vi "processCanFrame.vi"(1 "frame IN":u8[](array[numeric])) -> (0 "stateOut":enum16{"unconn", "reciving", "disconn"}(ring)=enum."reciving")   [LabVIEW 2021]
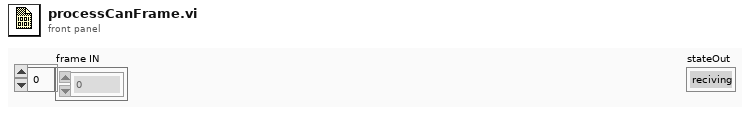
[diagram p1: front panel]
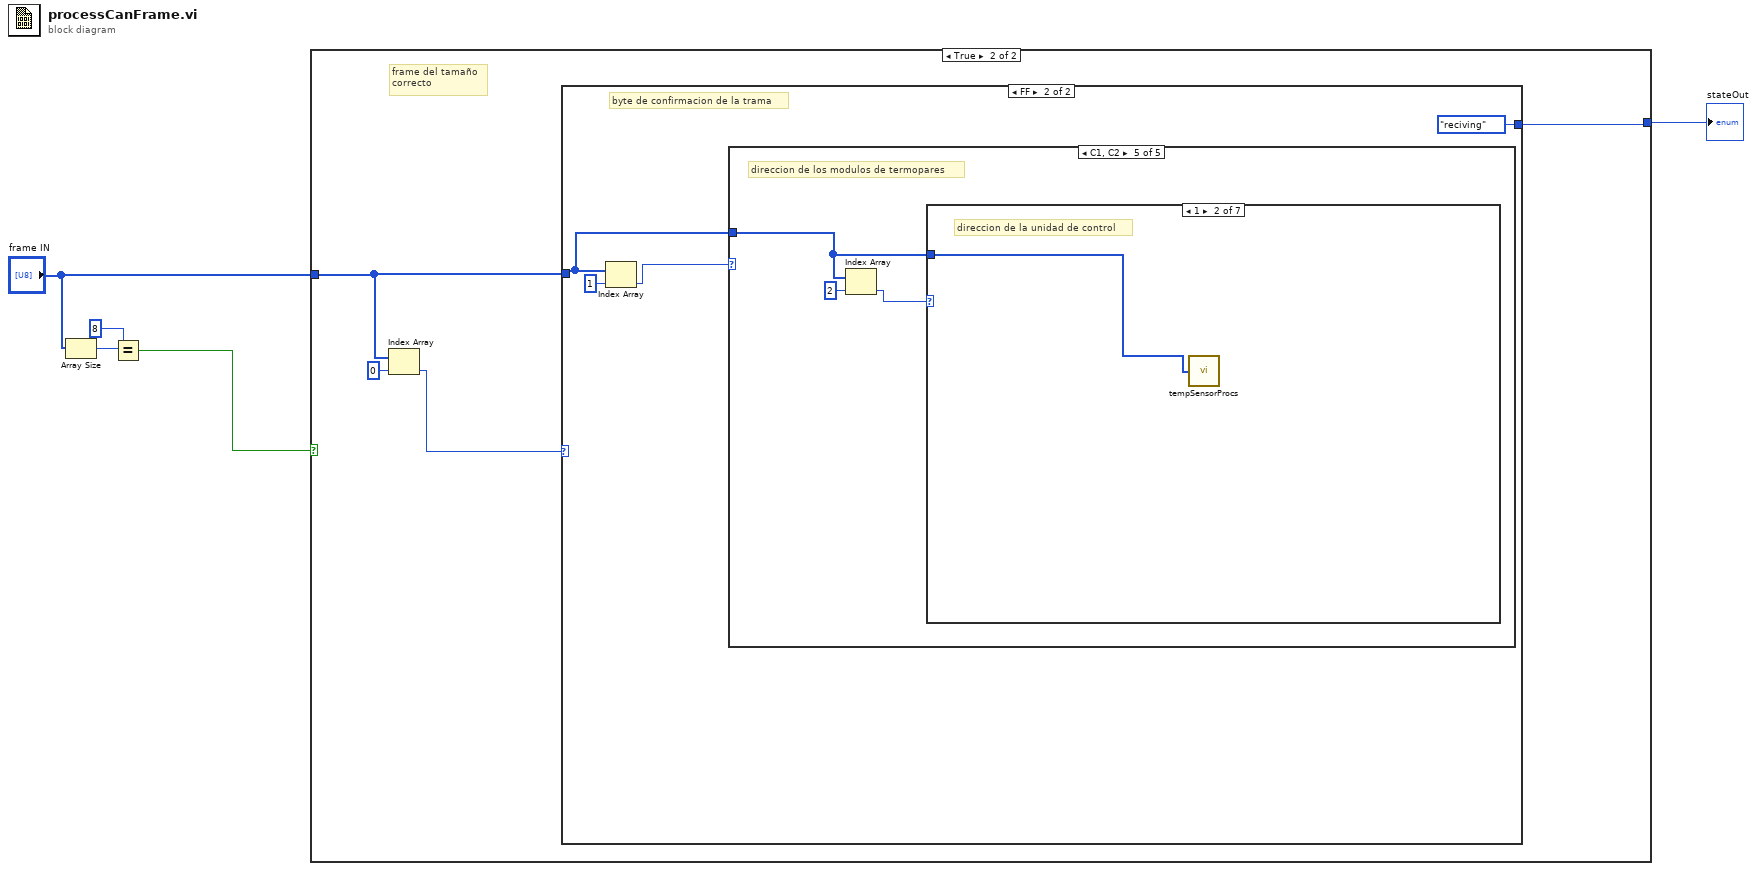
[diagram p0: block diagram]
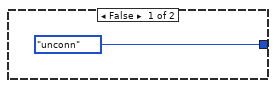
[diagram p2: hidden frame]
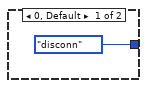
[diagram p3: hidden frame]
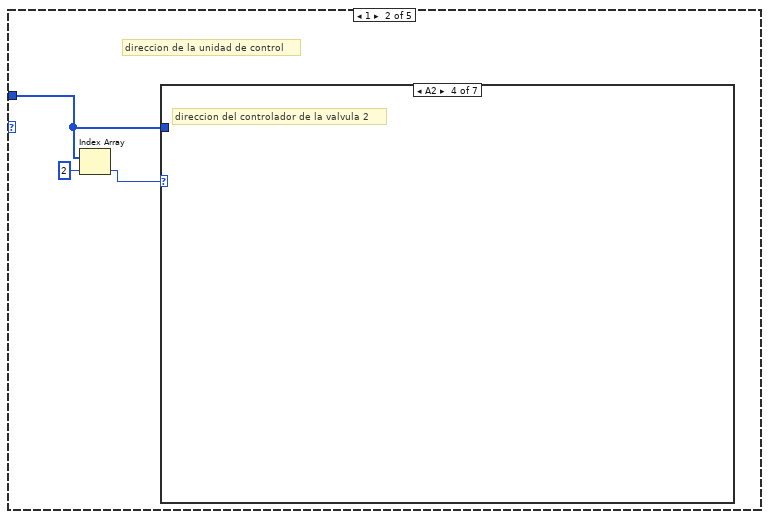
[diagram p5: hidden frame]
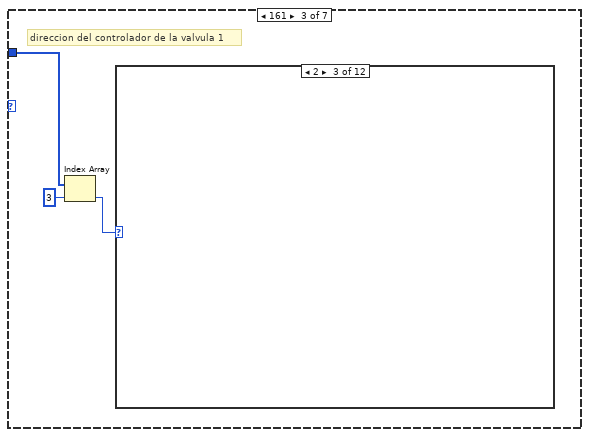
[diagram p8: hidden frame]
diagram:
  n1 = Array Size(array="frame IN") -> (size(s)=w4:i32)
  n2 = Equal?(x=w4, y=8) -> (x = y?=w2:bool)
  n3 = case shown="True" w2 {
    tunnel: "frame IN" -> [_ w9]
    tunnel: [enum16{"unconn", "reciving", "disconn"}."unconn" w7] -> w1
    frame False {
    }
    frame True {
      # "frame del tamaño\ncorrecto"
      n4 = Index Array(array=w9, index=0) -> (element=w8:u8)
      n5 = case shown="FF" w8 {
        tunnel: w9 -> [_ w13]
        tunnel: [enum16{"unconn", "reciving", "disconn"}."disconn" enum16{"unconn", "reciving", "disconn"}."reciving"] -> w7
        frame 0, Default {
        }
        frame 255 {
          # "byte de confirmacion de la trama"
          n6 = Index Array(array=w13, index=1) -> (element=w14:u8)
          n7 = case shown="C1, C2" w14 {
            tunnel: w13 -> [_ w16 w22 w29 w33]
            frame 0, Default {
            }
            frame 1 {
              # "direccion de la unidad de control"
              n8 = Index Array(array=w16, index=2) -> (element=w17:u8)
              n9 = case shown="A2" w17 {
                tunnel: w16 -> [_ _ w20 _ _ _ _]
                frame 0, Default {
                }
                frame 1 {
                  # "direccion de la unidad de control"
                }
                frame 161 {
                  # "direccion del controlador de la valvula 1"
                  n10 = Index Array(array=w20, index=3) -> (element=w19:u8)
                  n11 = case shown="2" w19 {
                    frame 0 {
                    }
                    frame 1 {
                    }
                    frame 2 {
                    }
                    frame 3 {
                    }
                    frame 4 {
                    }
                    frame 5 {
                    }
                    frame 6 {
                    }
                    frame 7 {
                    }
                    frame 8 {
                    }
                    frame 9 {
                    }
                    frame 10 {
                    }
                    frame 11, Default {
                    }
                  }
                }
                frame 162 {
                  # "direccion del controlador de la valvula 2"
                }
                frame 177 {
                  # "direccion del modulo de sensores de presion"
                }
                frame 193 {
                  # "direccion del modulo de termopares 1"
                }
                frame 194 {
                  # "direccion del modulo de termopares 2"
                }
              }
            }
            frame 161, 162 {
              # "direccion de los controladores de las valvulas"
              n12 = Index Array(array=w22, index=2) -> (element=w23:u8)
              n13 = case shown="1" w23 {
                tunnel: w22 -> [_ w25 _ _ _ _ _]
                frame 0, Default {
                }
                frame 1 {
                  # "direccion de la unidad de control"
                  n14 = Index Array(array=w25, index=3) -> (element=w26:u8)
                  n15 = case shown="4" w26 {
                    tunnel: w25 -> [_ w28]
                    frame 0, Default {
                    }
                    frame 4 {
                      n16 = call "valveDataProc.vi"("frame"=w28) -> ()
                    }
                  }
                }
                frame 161 {
                  # "direccion del controlador de la valvula 1"
                }
                frame 162 {
                  # "direccion del controlador de la valvula 2"
                }
                frame 177 {
                  # "direccion del modulo de sensores de presion"
                }
                frame 193 {
                  # "direccion del modulo de termopares 1"
                }
                frame 194 {
                  # "direccion del modulo de termopares 2"
                }
              }
            }
            frame 177 {
              # "direccion del modulo de sensores de presion"
              n17 = Index Array(array=w29, index=2) -> (element=w30:u8)
              n18 = case shown="1" w30 {
                tunnel: w29 -> [_ w32 _ _ _ _ _]
                frame 0, Default {
                }
                frame 1 {
                  # "direccion de la unidad de control"
                  n19 = call "pressSensorLin.vi"("frame"=w32) -> ()
                }
                frame 161 {
                  # "direccion del controlador de la valvula 1"
                }
                frame 162 {
                  # "direccion del controlador de la valvula 2"
                }
                frame 177 {
                  # "direccion del modulo de sensores de presion"
                }
                frame 193 {
                  # "direccion del modulo de termopares 1"
                }
                frame 194 {
                  # "direccion del modulo de termopares 2"
                }
              }
            }
            frame 193, 194 {
              # "direccion de los modulos de termopares"
              n20 = Index Array(array=w33, index=2) -> (element=w34:u8)
              n21 = case shown="1" w34 {
                tunnel: w33 -> [_ w36 _ _ _ _ _]
                frame 0, Default {
                }
                frame 1 {
                  # "direccion de la unidad de control"
                  n22 = call "tempSensorProcs.vi"("frame"=w36) -> ()
                }
                frame 161 {
                  # "direccion del controlador de la valvula 1"
                }
                frame 162 {
                  # "direccion del controlador de la valvula 2"
                }
                frame 177 {
                  # "direccion del modulo de sensores de presion"
                }
                frame 193 {
                  # "direccion del modulo de termopares 1"
                }
                frame 194 {
                  # "direccion del modulo de termopares 2"
                }
              }
            }
          }
        }
      }
    }
  }
  "stateOut" <- w1
